vi "8PSK (SubVI) .vi"(11 "output bit stream":i8[](array[numeric])) -> (3 "Array":cdb[](array[numeric]))   [LabVIEW 2018]
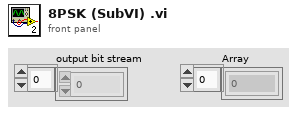
[diagram p1: front panel]
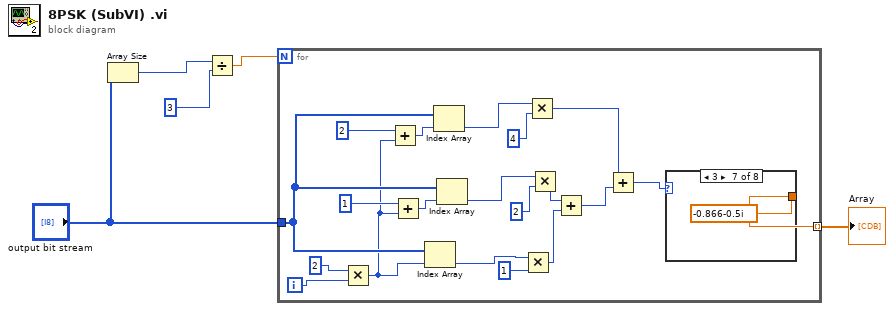
[diagram p0: block diagram]
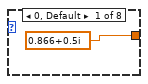
[diagram p2: hidden frame]
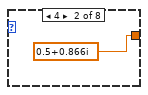
[diagram p3: hidden frame]
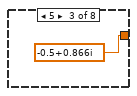
[diagram p4: hidden frame]
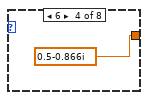
[diagram p5: hidden frame]
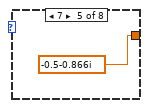
[diagram p6: hidden frame]
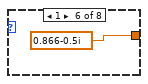
[diagram p7: hidden frame]
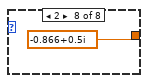
[diagram p8: hidden frame]
diagram:
  n1 = Array Size(array="output bit stream") -> (size(s)=w2:i32)
  n2 = Divide(x=w2, y=3) -> (x/y=w4:dbl)
  n3 = for {
    N: w4 -> [_]
    tunnel: "output bit stream" -> [w10]
    tunnel: [w15] -> w5 mode=indexing
    i -> [w22]
    n4 = Multiply(x=2, y=w22) -> (x*y=w9:i32)
    n5 = Add(x=2, y=w9) -> (x+y=w14:i32)
    n6 = Add(x=1, y=w9) -> (x+y=w25:i32)
    n7 = Index Array(array=w10, index=w9) -> (element=w18:i8)
    n8 = Index Array(array=w10, index=w14) -> (element=w11:i8)
    n9 = Index Array(array=w10, index=w25) -> (element=w20:i8)
    n10 = Multiply(x=w18, y=1) -> (x*y=w16:i32)
    n11 = Multiply(x=w11, y=4) -> (x*y=w8:i32)
    n12 = Multiply(x=w20, y=2) -> (x*y=w17:i32)
    n13 = Add(x=w17, y=w16) -> (x+y=w7:i32)
    n14 = Add(x=w8, y=w7) -> (x+y=w6:i32)
    n15 = case shown="3" w6 {
      tunnel: [cdb 0.866+0.5i cdb 0.5+0.866i cdb -0.5+0.866i cdb 0.5-0.866i cdb -0.5-0.866i cdb 0.866-0.5i cdb -0.866-0.5i cdb -0.866+0.5i] -> w15
      frame 0, Default {
      }
      frame 4 {
      }
      frame 5 {
      }
      frame 6 {
      }
      frame 7 {
      }
      frame 1 {
      }
      frame 3 {
      }
      frame 2 {
      }
    }
  }
  "Array" <- w5
